vi "AAL Error Information.vi"(8 "error in (no error)":errorcluster, 11 "error code":i32) -> (0 "error out":errorcluster)   [LabVIEW 2018, in "NI_AALPro.lvlib"]
uses:
  NI_AALPro.lvlib
panel:
  # "Error Information"
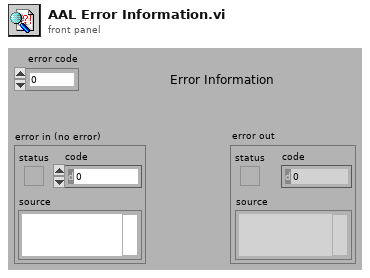
[diagram p1: front panel]
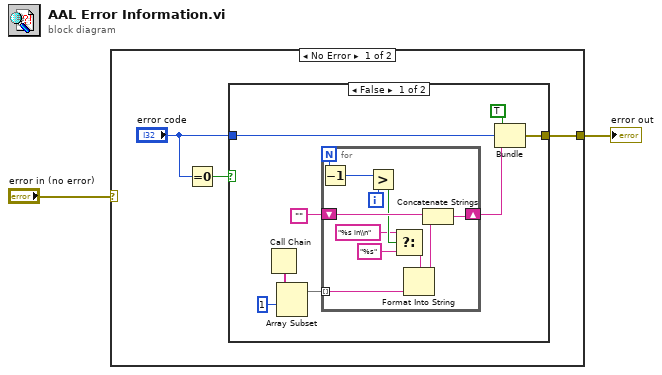
[diagram p0: block diagram]
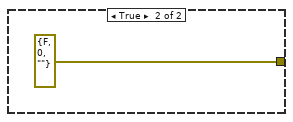
[diagram p2: hidden frame]
diagram:
  n1 = case shown="No Error" "error in (no error)" {
    selector: "error in (no error)" -> [_ w26]
    tunnel: [w3 w26] -> w1
    frame No Error {
      n2 = Equal To 0?(x="error code") -> (x = 0?=w5:bool)
      n3 = case shown="False" w5 {
        tunnel: "error code" -> [w6 _]
        tunnel: [w7 errorcluster {"status"=FALSE, "code"=0, "source"=""} ("error out")] -> w3
        frame False {
          n4 = Call Chain() -> (call chain=w10:string[])
          n5 = Array Subset(array=w10, index=1) -> (w11:string[])  [unwired: 1 in]
          n6 = for {
            N -> [w19]
            shift-right: [w23] -> w8
            shift-left: "" -> [w24]
            tunnel: w11 -> [w17] mode=indexing
            i -> [w18]
            n7 = Decrement(x=w19) -> (x-1=w20:i32)
            n8 = Greater?(x=w20, y=w18) -> (0:w21:bool)
            n9 = Select(t="%s in\\n", s=w21, f="%s") -> (s? t:f=w14:string)
            n10 = Format Into String(format string=w14, w17) -> (resulting string=w22:string)  [unwired: 2 in, 1 out]
            n11 = Concatenate Strings(w24, w22) -> (w23:string)
          }
          n12 = Bundle(TRUE, "error code"=w6, w8) -> (w7:cluster{bool, "error code":i32, string})  [unwired: 1 in]
        }
        frame True {
        }
      }
    }
    frame Error {
    }
  }
  "error out" <- w1
